vi "statusLEDs_read.vi"(3 "error in (no error)":errorcluster, 5 "SCI":u8) -> (0 "Error Out":errorcluster)   [LabVIEW 2013]
uses:
  My Computer/Controls/Sepios_status.ctl
panel:
  out "initialized array":u16[][](array[numeric])
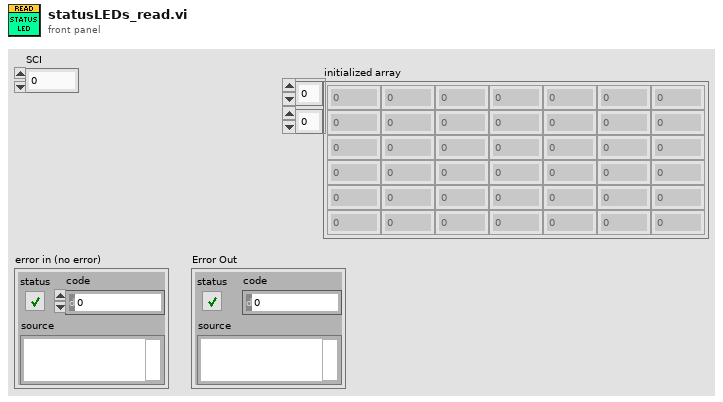
[diagram p1: front panel]
types:
  T1 = typedef "Sepios_status.ctl" = enum16{"Standby", "Running", "Filming", "Error"}
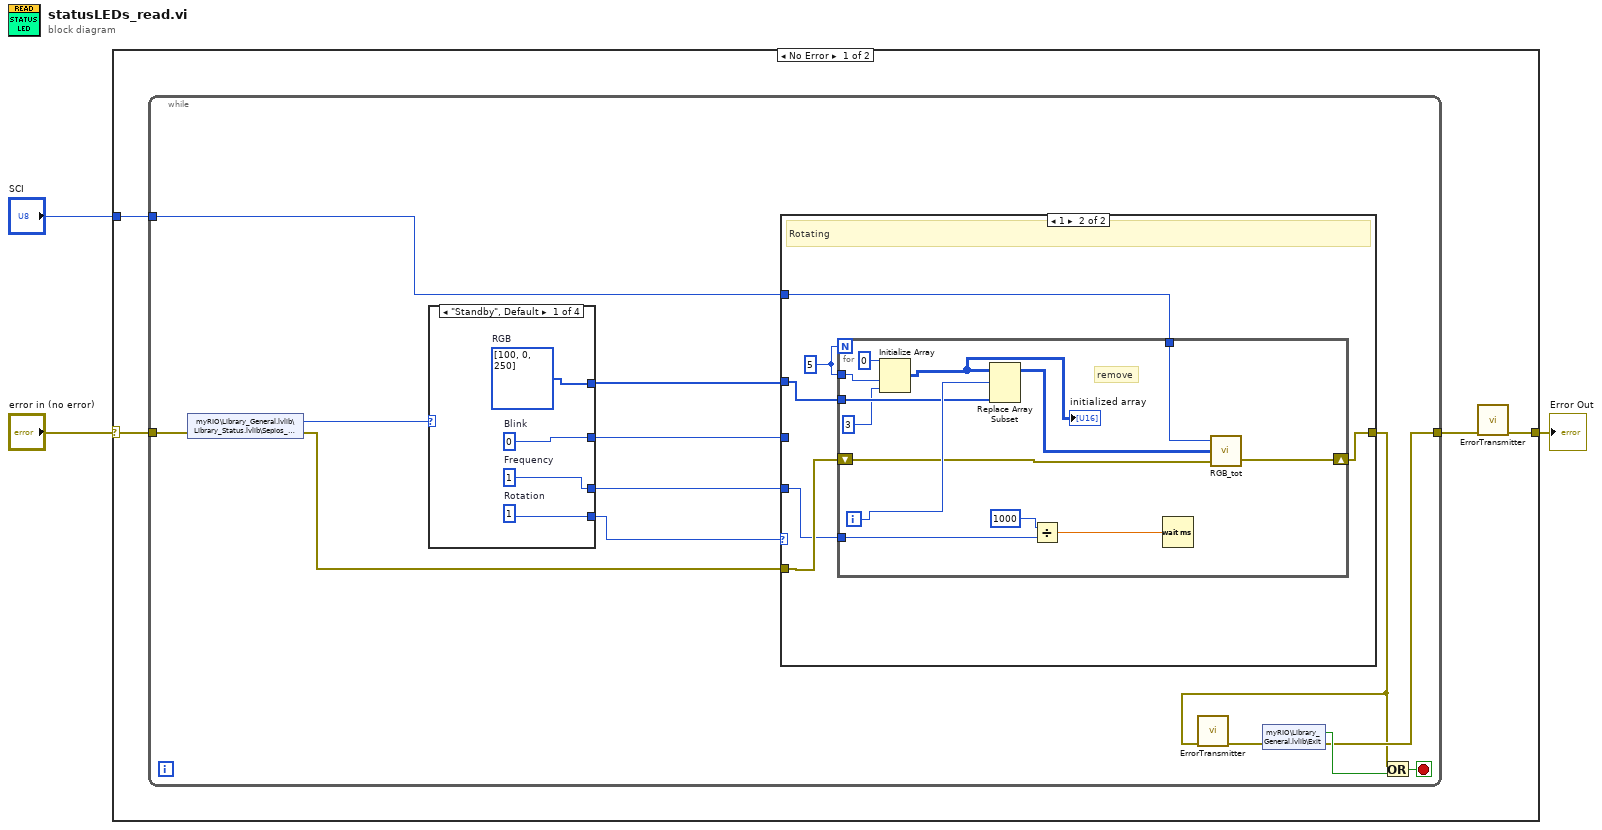
[diagram p0: block diagram]
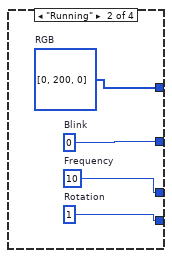
[diagram p2: hidden frame]
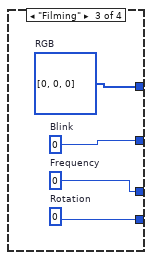
[diagram p3: hidden frame]
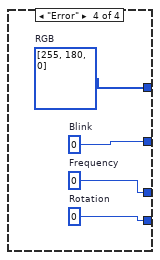
[diagram p4: hidden frame]
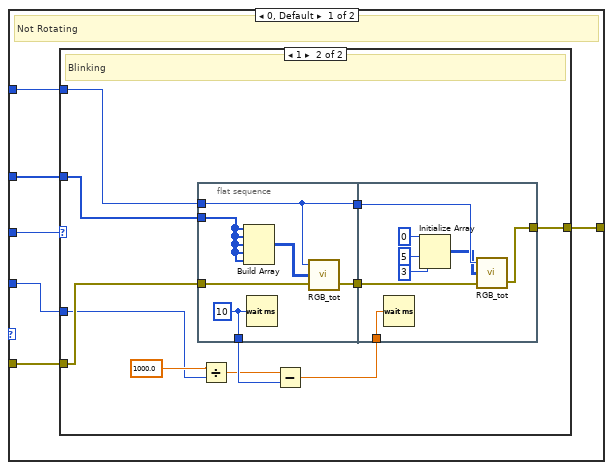
[diagram p5: hidden frame]
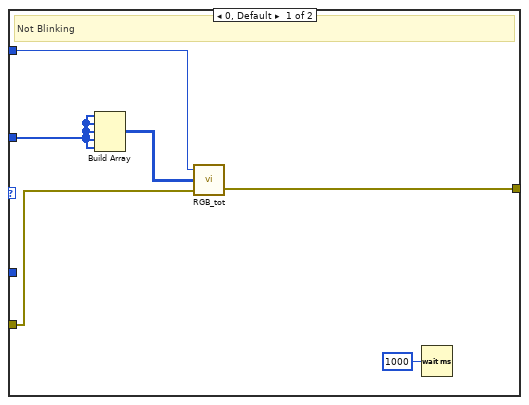
[diagram p6: hidden frame]
diagram:
  n1 = case shown="No Error" "error in (no error)" {
    selector: "error in (no error)" -> [w4 w93]
    tunnel: "SCI" -> [w7 _]
    tunnel: [w5 w93] -> w2
    frame No Error {
      n2 = while {
        tunnel: w4 -> [w19]
        tunnel: w7 -> [w18]
        tunnel: [w10] -> w6
        stop <- w11 stop-if-true
        n3 = shared-variable "myRIO\\Library_General.lvlib\\Library_Status.lvlib\\Sepios_Status"(error in=w19) -> (w13:T1, error out=w20:errorcluster)
        n4 = case shown="\"Standby\", Default" w13 {
          tunnel: [w21 w25 w29 w33] -> w17
          tunnel: [w24 w28 w32 w36] -> w16
          tunnel: [w23 w27 w31 w35] -> w15
          tunnel: [w22 w26 w30 w34] -> w14
          frame "Standby", Default {
            w21 = u16[] [100, 0, 250]  # RGB
            w22 = u16 1  # Rotation
            w23 = u16 1  # Frequency
            w24 = u16 0  # Blink
          }
          frame "Running" {
            w25 = u16[] [0, 200, 0]  # RGB
            w26 = u16 1  # Rotation
            w27 = u16 10  # Frequency
            w28 = u16 0  # Blink
          }
          frame "Filming" {
            w29 = u16[] [0, 0, 0]  # RGB
            w30 = u16 0  # Rotation
            w31 = u16 0  # Frequency
            w32 = u16 0  # Blink
          }
          frame "Error" {
            w33 = u16[] [255, 180, 0]  # RGB
            w34 = u16 0  # Rotation
            w35 = u16 0  # Frequency
            w36 = u16 0  # Blink
          }
        }
        n5 = case shown="1" w14 {
          tunnel: w16 -> [w42 _]
          tunnel: w15 -> [w39 w74]
          tunnel: w18 -> [w41 w77]
          tunnel: w17 -> [w40 w76]
          tunnel: [w38 w78] -> w9
          tunnel: w20 -> [w37 w75]
          frame 0, Default {
            # "Not Rotating"
            n6 = case shown="1" w42 {
              tunnel: [w47 w59] -> w38
              tunnel: w41 -> [w48 w57]
              tunnel: w40 -> [w44 w58]
              tunnel: w39 -> [_ w52]
              tunnel: w37 -> [w46 w56]
              frame 0, Default {
                # "Not Blinking"
                n7 = Build Array(w44, w44, w44, w44, w44) -> (w43:u16[][])
                n8 = call "RGB_tot.vi"("error in"=w46, "output array"=w43, "SCI"=w48) -> ("error out"=w47:errorcluster)  [unwired: 1 in]
                n9 = Wait (ms)(milliseconds to wait=u32 1000) -> ()  [unwired: 1 out]
              }
              frame 1 {
                # "Blinking"
                n10 = flat-sequence {
                  tunnel: w57 -> [w65]
                  tunnel: w58 -> [w62]
                  tunnel: [w65] -> w55
                  tunnel: [w64] -> w54
                  tunnel: w56 -> [w63]
                  tunnel: [w60] -> w51
                  tunnel: [w73] -> w59
                  tunnel: w55 -> [w72]
                  tunnel: w54 -> [w71]
                  tunnel: w49 -> [w70]
                  frame #0 {
                    w60 = u32 10 ("milliseconds to wait")
                    n11 = Build Array(w62, w62, w62, w62, w62) -> (w61:u16[][])
                    n12 = Wait (ms)(milliseconds to wait=w60) -> ()  [unwired: 1 out]
                    n13 = call "RGB_tot.vi"("error in"=w63, "output array"=w61, "SCI"=w65) -> ("error out"=w64:errorcluster)  [unwired: 1 in]
                  }
                  frame #1 {
                    n14 = Wait (ms)(milliseconds to wait=w70) -> ()  [unwired: 1 out]
                    n15 = Initialize Array(u16 0 ("element"), 5 ("dimension size"), 3 ("dimension size")) -> (w67:u16[][])
                    n16 = call "RGB_tot.vi"("error in"=w71, "output array"=w67, "SCI"=w72) -> ("error out"=w73:errorcluster)  [unwired: 1 in]
                  }
                }
                n17 = Divide(x=1000.0 ("y"), y=w52) -> (x/y=w50:dbl)
                n18 = Subtract(x=w50, y=w51) -> (x-y=w49:dbl)
              }
            }
          }
          frame 1 {
            w79 = 5 ("dimension size")
            # "Rotating"
            n19 = for {
              N: w79 -> [_]
              tunnel: w79 -> [w84]
              tunnel: w76 -> [w89]
              tunnel: w77 -> [w88]
              shift-right: [w85] -> w78
              shift-left: w75 -> [w86]
              tunnel: w74 -> [w80]
              i -> [w91]
              # "remove"
              n20 = Initialize Array(u16 0 ("element"), w84, 3 ("dimension size")) -> (w90:u16[][])
              "initialized array" <- w90
              n21 = Replace Array Subset(array=w90, new element=w89, index (row)=w91) -> (w87:u16[][])  [unwired: 1 in]
              n22 = Divide(x=1000, y=w80) -> (x/y=w82:dbl)
              n23 = Wait (ms)(milliseconds to wait=w82) -> ()  [unwired: 1 out]
              n24 = call "RGB_tot.vi"("error in"=w86, "output array"=w87, "SCI"=w88) -> ("error out"=w85:errorcluster)  [unwired: 1 in]
            }
          }
        }
        n25 = call "ErrorTransmitter.vi"("Error In"=w9) -> ("Error Out"=w8:errorcluster)  [unwired: 10 in]
        n26 = shared-variable "myRIO\\Library_General.lvlib\\Exit"(error in=w8) -> (w12:bool, error out=w10:errorcluster)
        n27 = Or(x=w9, y=w12) -> (x .or. y?=w11:bool)
      }
      n28 = call "ErrorTransmitter.vi"("Error In"=w6) -> ("Error Out"=w5:errorcluster)  [unwired: 10 in]
    }
    frame Error {
    }
  }
  "Error Out" <- w2
